vi "Destroy DSF Configuration Session.vi"(8 "error in (no error)":errorcluster, 11 "DSF Configuration Session in":T1) -> (0 "error out":errorcluster)   [LabVIEW 2017, in "DSF Configuration API.lvlib"]
uses:
  DSF Configuration API.lvlib
  Controls/Session/DSF Configuration Reference.ctl
  Controls/Session/Config Data.ctl
  Controls/DSF File Format/DSF Configuration with ID.ctl
  Public/Controls/DSF Version Info.ctl
  Controls/DSF File Format/DSF Plugin with ID.ctl
  Public/Controls/DSF Plugin Info.ctl
  Public/Controls/DSF Timing Info.ctl
  Controls/DSF File Format/DSF Group with ID.ctl
  Public/Controls/DSF Group Info.ctl
  Controls/DSF File Format/DSF Transfer with ID.ctl
  Public/Controls/DSF Transfer Info.ctl
  Controls/DSF File Format/DSF Channel with ID.ctl
  Public/Controls/DSF Channel Info.ctl
  Controls/DSF File Format/DSF Settings with ID.ctl
  Public/Controls/DSF Settings Info.ctl
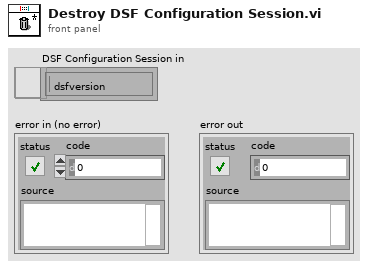
[diagram p1: front panel]
types:
  T1 = typedef "DSF Configuration API.lvlib/DSF Configuration Reference.ctl" = refnum<data-value>
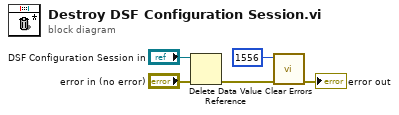
[diagram p0: block diagram]
diagram:
  n1 = Delete Data Value Reference(data value reference="DSF Configuration Session in", error in="error in (no error)") -> (error out=w5:errorcluster)  [unwired: 1 out]
  n2 = call <vilib>:"Clear Errors.vi"("error in (no error)"=w5, "specific error code to clear (0: all)"=1556) -> ("error out"=→"error out":errorcluster)  [unwired: 4 in, 1 out]
